vi "svl_Log View for Energy Level (N Ch) (single value).vi"(7 "waveform parameters":waveform(dbl)[](array[waveform]), 8 "error in (no error)":errorcluster, 9 "view mode":enum16{"Power", "Amplitude"}(ring), 10 "dB On (T)":bool=TRUE, 11 "energy levels [EU^2 rms]":dbl[](array[numeric]) format="%.2f") -> (0 "error out":errorcluster, 2 "unit label [ ]":string[](array[string]), 3 "energy levels [EU^2 rms]":dbl[](array[numeric]) format="%.2f")   [LabVIEW 2017]
uses:
  <vilib>/addons/_NISVFA/_Shared subVIs/Common/svc_Engineering Units to Unit Label.vi
  <vilib>/addons/_NISVFA/_Shared subVIs/Common/svc_Unit Label to Engineering Units.vi
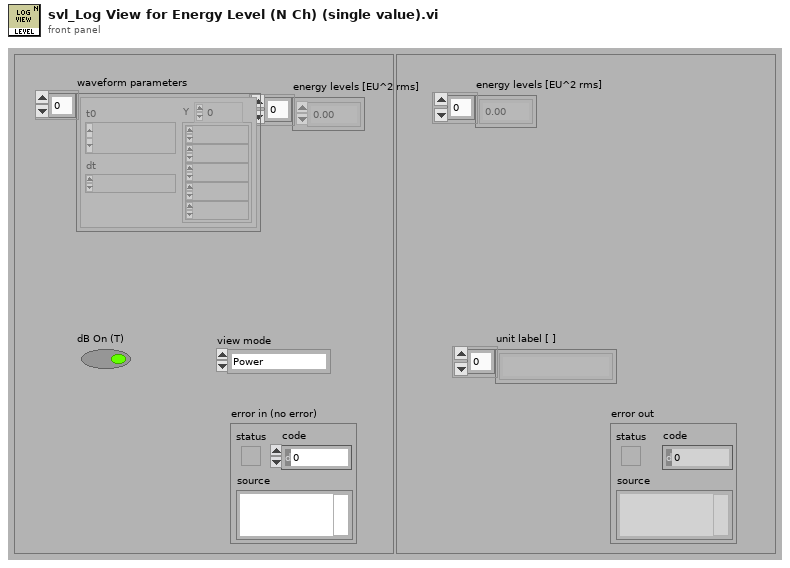
[diagram p1: front panel]
types:
  T1 = typedef "svc_Channel Info.ctl" = cluster{"sensor sensitivity":dbl, "engineering units":T2, "dB reference":dbl, "custom label":string, "weighting filter":T3, "pregain":dbl}
  T2 = typedef "svc_Engineering Units Text Ring.ctl" = u16
  T3 = typedef "svc_Weighting Filter Text Ring.ctl" = u16
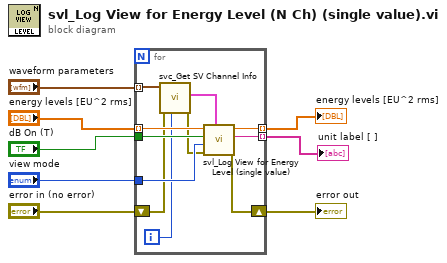
[diagram p0: block diagram]
diagram:
  n1 = for {
    tunnel: "energy levels [EU^2 rms]" -> [w18] mode=indexing
    tunnel: "dB On (T)" -> [w16]
    tunnel: "waveform parameters" -> [w13] mode=indexing
    tunnel: [w17] -> w6 mode=indexing
    tunnel: [w15] -> w5 mode=indexing
    shift-right: [w19] -> w2
    shift-left: "error in (no error)" -> [w11]
    tunnel: "view mode" -> [w14]
    i -> [w9]
    n2 = call <vilib>:"svc_Get SV Channel Info.vi"("channel index"=w9, "error in (no error)"=w11, "scaled signal [EU]"=w13) -> ("error out"=w10:errorcluster, "channel info"=w12:T1)  [unwired: 3 in, 4 out]
    n3 = call <vilib>:"svl_Log View for Energy Level (single value).vi"("channel info"=w12, "error in (no error)"=w10, "view mode"=w14, "dB On (T)"=w16, "energy level [EU^2 rms]"=w18) -> ("error out"=w19:errorcluster, "unit label"=w15:string, "energy level [EU^2 rms]"=w17:dbl)  [unwired: 4 in]
  }
  "unit label [ ]" <- w5
  "energy levels [EU^2 rms]" <- w6
  "error out" <- w2
